vi "GetFirstDeviceKey_8742.vi"(4 "error in":errorcluster, 7 "CmdLib In":refnum<k24>) -> (0 "error out":errorcluster, 2 "DeviceKey Out":string, 3 "CmdLib Out":refnum<k24>)   [LabVIEW 2009]
uses:
  C:/Code/Apps/Utilities/Picomotor/PicomotorApp/Install/Samples/LabVIEW/Mixed Devices/LabVIEW 2009/CmdLib8742.dll
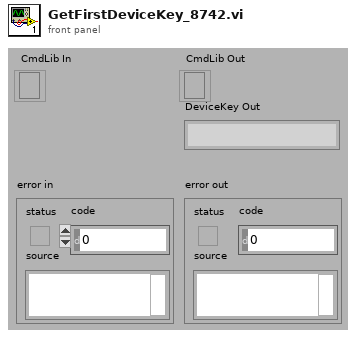
[diagram p1: front panel]
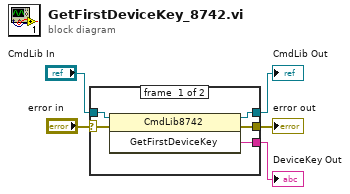
[diagram p0: block diagram]
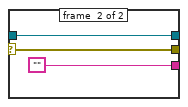
[diagram p2: hidden frame]
diagram:
  n1 = case shown="No Error" "error in" {
    selector: "error in" -> [w7 w13]
    tunnel: "CmdLib In" -> [w10 w11]
    tunnel: [w9 ""] -> w4
    tunnel: [w8 w13] -> w3
    tunnel: [w6 w11] -> w1
    frame #0 {
      n2 = invoke class="CmdLib8742" method="GetFirstDeviceKey"(reference=w10, error in=w7) -> (reference out=w6:refnum<k24>, error out=w8:errorcluster, "GetFirstDeviceKey"=w9:string)  [unwired: 1 in]
    }
    frame #1 {
    }
  }
  "DeviceKey Out" <- w4
  "error out" <- w3
  "CmdLib Out" <- w1
